vi "STA - Wave V5 Host_Wait_V4.vi"() -> ()   [LabVIEW 2015]
doc: "The continuous acquisition mode tells the FPGA to acquire points indefinitely until a stop command is issued or until an error is encountered (FIFO overflow, module underflow, and so on). \n\nIn this acquisition mode, explicitly call the appropriate rwfm_ConfigTiming VI and set the host application's data buffer to be many times larger than the read size. The examples use a 10X size by default. If the host application's data buffer fills, then the FPGA experiences a FIFO overflow causing the acquisition to stop."
uses:
  <vilib>/LabVIEW Targets/FPGA/cRIO/shared/nicrio_ModuleControls/nicrio_cRIO-9234_ConfigModeRing.ctl
  <vilib>/Platform/TimedLoop/XDataNode/timing_clust.ctl
  <vilib>/Platform/TimedLoop/XDataNode/nitl_modes.ctl
  <vilib>/Platform/TimedLoop/XDataNode/wakeup.ctl
  <vilib>/FPGAPlugInAG/cRIO-9112/niLvFpga_Open_cRIO-9112.vi
  <vilib>/rvi/interface/common/dynamic/niFpgaDynamicAddResources.vi
  <vilib>/Utility/error.llb/Error Cluster From Error Code.vi
  <vilib>/RVI Host/nirviSupport.llb/nirviErrorClusterFromErrorCode.vi
  <vilib>/rvi/errors/niLvFpgaAdjustHostInterfaceError.vi
  <vilib>/FPGAPlugInAG/Dynamic/niLvFpga_Close_Dynamic.vi
  <vilib>/NI/cRIO Wfm/AcqRead(InterleavedSGLs).vi
  <vilib>/rvi/interface/nirviOpenFPGA/nirviOpenFPGA.xnode
  FPGA Bitfiles/STA-WaveformV5_FPGATarget2_[FPGA]DeltaSigMa_sLRIAVfzKK0.lvbitx
  FPGA/[FPGA] DeltaSig Main V5.vi
  <vilib>/rvi/interface/nirviMethod/nirviMethod.xnode
  <vilib>/rvi/interface/nirviCloseFPGA/nirviCloseFPGA.xnode
  <vilib>/Platform/TimedLoop/XDataNode/XDataNode.xnode
  <vilib>/NI/cRIO Wfm/cRIO Wfm.lvlib
  <vilib>/rvi/interface/nirviMethod/StockFPGA_InlinedMethodWaitForSingleIRQ.vi
  <vilib>/FPGAPlugInAG/Dynamic/niLvFpga_WaitOnIrq_Dynamic.vi
  C:/Program Files (x86)/National Instruments/LabVIEW 2015/ProjectTemplates/Source/cRIOWfm/FPGA/[FPGA] SAR Acq Main.vi
  D/Documents/LabVIEW Data/STA - Waveform V0/FPGA Bitfiles/SARAcqMain_9074.lvbitx
  <vilib>/Platform/TimedLoop/XDataNode/XDNodeRunTimeDep.lvlib
panel:
  out "RT Read Side element":u32
  out "RT Write element":u32
  out "Write Side":sgl[][](array[numeric])
  out "transposed array Read Side":sgl[][](array[numeric])
  out "Loop i Read Side":i32
  in  "stop 2":bool
  out "element out Read Side":sgl[](array[numeric])
  out "Write Side out":sgl[](array[numeric])
  in  "Input RTFIFO Create":sgl[](array[numeric])
  in  "Wfm Data":waveform(sgl)[](array[waveform])
  out "Time Measure":dbl
  out "data rate (S/s)":u32
  out "Channel Config":T2(array[cluster]) {"Input Configuration" items=["AC Coupled", "DC Coupled", "IEPE AC Coupled"]}
  in  "Samples per Read":i32=10000
  in  "stop":bool
  out "Waveform Graph Read Side":sgl[](graph)
  out "Buffer Backlog":dbl caption="RT Buffer Backlog [%]" format="%#.2g"
  # "Sampling Info"
  # "Channel Info"
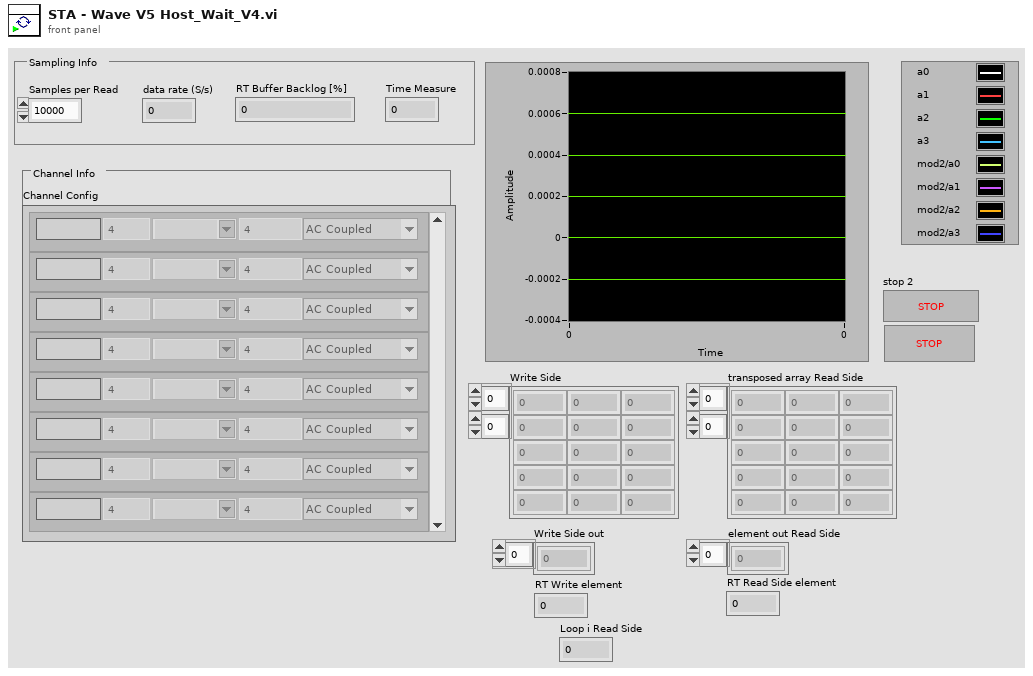
[diagram p1: front panel]
types:
  T1 = typedef "nicrio_cRIO-9234_ConfigModeRing.ctl" = u8
  T2 = cluster{"Channel Name":string, "Sensitivity mV_EU":dbl, "EU":string, "Input Configuration":T1, "dB Ref EU":dbl}[]
  T3 = typedef "XDNodeRunTimeDep.lvlib/timing_clust.ctl" = cluster{"Expected End [f-1]":u64, "Actual End [f-1]":u64, "Finished Late? [f-1]":bool, "Expected End [i-1]":u64, "Actual End [i-1]":u64, "Finished Late? [i-1]":bool, "Expected Start [i]":u64, "Actual Start [i]":u64, "Expected Start [f]":u64, "Actual Start [f]":u64, "Source Name":string, "Structure Name":string, "Period":i64, "Deadline":i64, "Offset":i64, "Start":i64, "Priority":i32, "Timeout":i32, "Mode":T4, "Wakeup Reason":T5, "Error":errorcluster, "Source Type":string, "Secondary Source Type":string, "Global End Time":u64, "Global Start Time":u64, "Frame Duration":u64, "Iteration Duration":u64, "Assigned CPU":i32, "I/O Scan Engine Mode":u32}
  T4 = typedef "XDNodeRunTimeDep.lvlib/nitl_modes.ctl" = enum32{"No Change", "Process missed periods, maintain original phase", "Discard missed periods, maintain original phase", "Process missed periods, ignore original phase", "Discard missed periods, ignore original phase"}
  T5 = typedef "XDNodeRunTimeDep.lvlib/wakeup.ctl" = enum32{"Normal", "Aborted", "Asynchronous wakeup", "Timing source error", "Timed loop error", "Timeout"}
  T6 = typedef "Acquisition and Logging Configuration_Waveform.ctl" = cluster{"Samples per Read":i32, "Number of Reads to Save":i32, "Data File Name":string, "TDMS Properties":T7[], "Number of Channels":i32, "Trigger - RMS Value":dbl, "Trigger - Channel":i32, "Trigger - Time (Minute)":i32, "Channel Config":cluster{"Channel Name":string, "Sensitivity mV_EU":dbl, "EU":string, "Input Configuration":T1, "dB Ref EU":dbl}[], "data rate (S/s)":u32, "Time Measure":dbl}
  T7 = typedef "TDMS Properties.ctl" = cluster{"Name":string, "Value":string}
  T8 = typedef "cRIO Wfm.lvlib/SamplingInfo.ctl" = cluster{"Number of Channels":i32, "Actual Samp Rate":dbl, "Chan Name Array":string[], "EU Chan Array":string[], "dB Ref Chan Array":dbl[]}
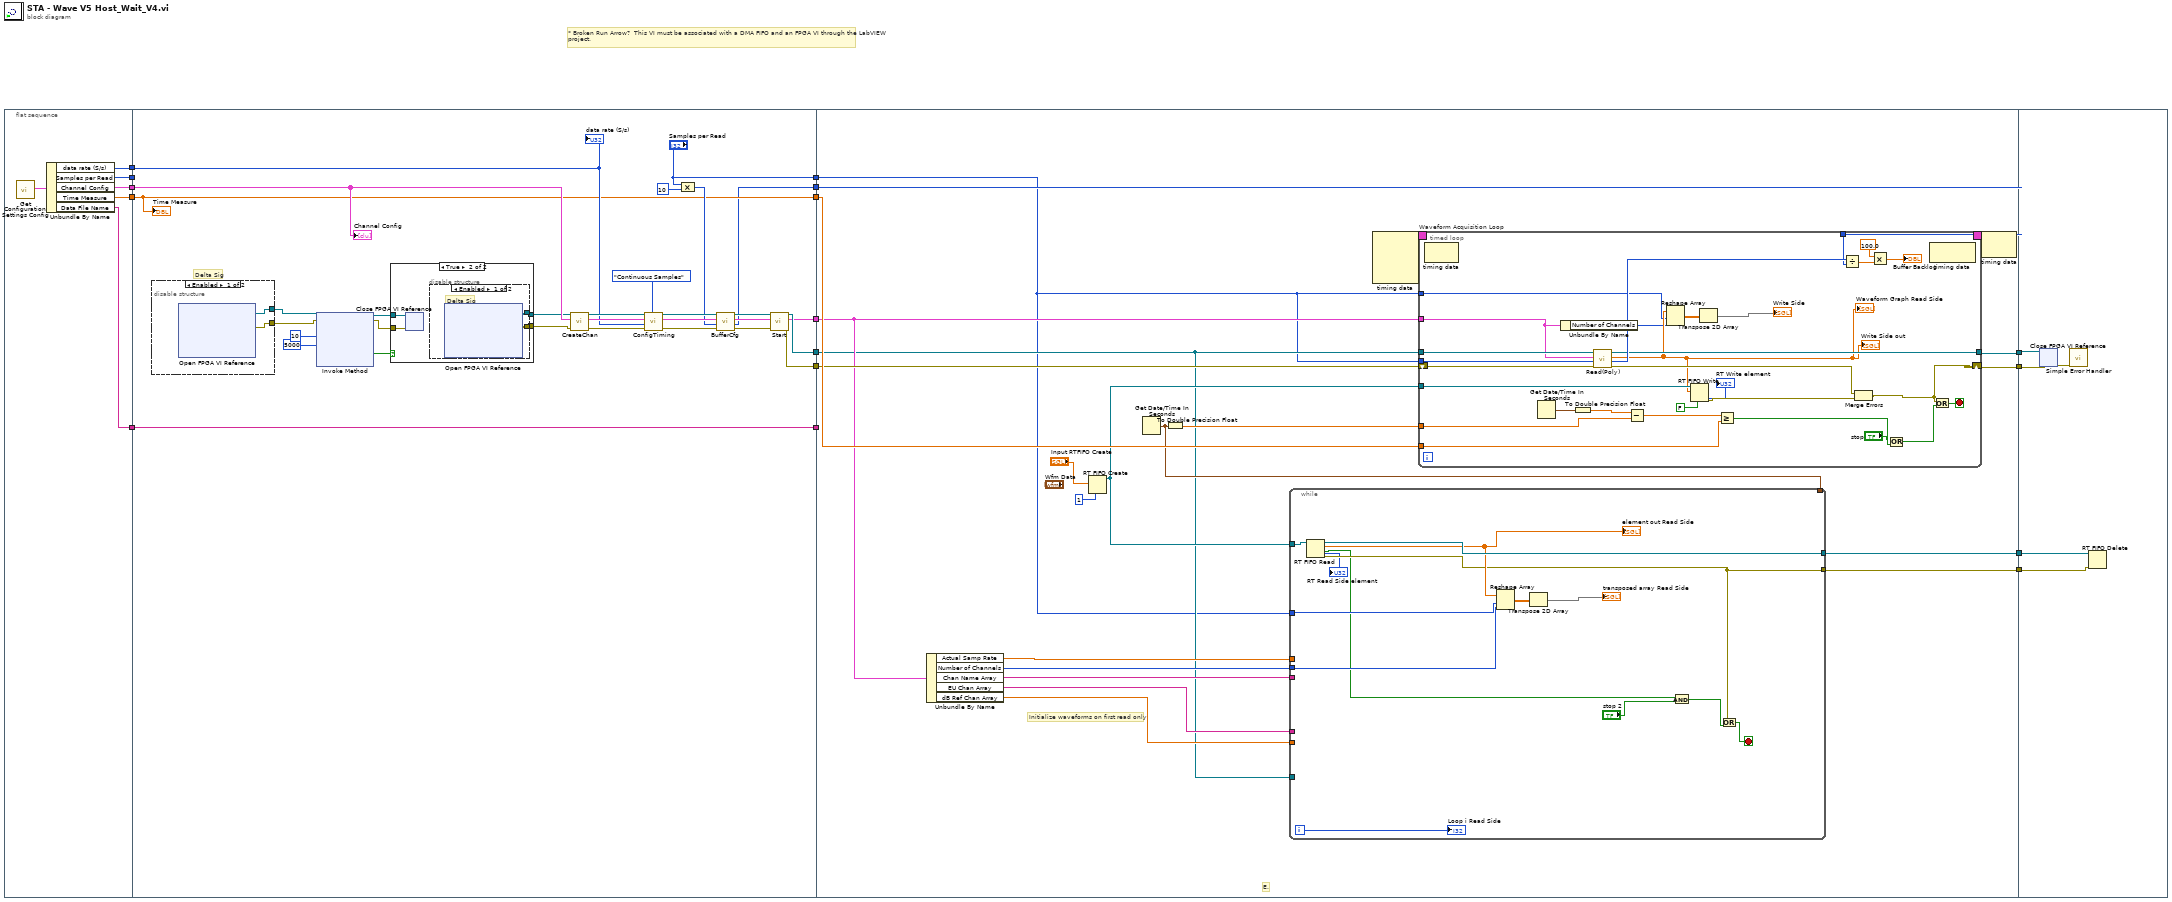
[diagram p0: block diagram]
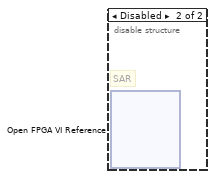
[diagram p2: hidden frame]
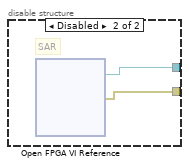
[diagram p4: hidden frame]
diagram:
  # "* Broken Run Arrow?  This VI must be associated with a DMA FIFO and an FPGA VI through the LabVIEW project."
  n1 = flat-sequence {
    tunnel: [w21] -> w16
    tunnel: [w20] -> w15
    tunnel: [w19] -> w14
    tunnel: [w18] -> w13
    tunnel: [w17] -> w4
    tunnel: w16 -> [w34]
    tunnel: w15 -> [_]
    tunnel: w14 -> [w33]
    tunnel: w13 -> [w26]
    tunnel: ["Samples per Read"] -> w12
    tunnel: [w26] -> w11
    tunnel: [w30] -> w10
    tunnel: [w29] -> w9
    tunnel: [w28] -> w8
    tunnel: [w25] -> w7
    tunnel: w4 -> [w24]
    tunnel: [w24] -> w3
    tunnel: w12 -> [w67]
    tunnel: w11 -> [w85]
    tunnel: w10 -> [w68]
    tunnel: w9 -> [w70]
    tunnel: w8 -> [w83]
    tunnel: w7 -> [w84]
    tunnel: [w87] -> w6
    tunnel: [w86] -> w5
    tunnel: w3 -> [_]
    tunnel: [w78] -> w2
    tunnel: [w77] -> w1
    tunnel: w6 -> [w140]
    tunnel: w5 -> [w139]
    tunnel: w2 -> [w138]
    tunnel: w1 -> [w137]
    frame #0 {
      n2 = call "Get Configuration Settings Config.vi"() -> ("Configuration"=w22:T6)  [unwired: 10 in, 1 out]
      n3 = Unbundle By Name(w22) -> ("data rate (S/s)"=w21:u32, "Samples per Read"=w20:i32, "Channel Config"=w19:T2, "Time Measure"=w18:dbl, "Data File Name"=w17:string)
    }
    frame #1 {
      # "Delta Sig"
      n4 = disable-structure shown="Enabled" {
        disable-tunnel: [w54 _] -> w32
        disable-tunnel: [w53 _] -> w31
        frame Enabled {
          n5 = xnode "Open FPGA VI Reference"() -> ("FPGA VI Reference Out"=w54:refnum<k20>, "error out"=w53:errorcluster)  [unwired: 2 in]
        }
        frame Disabled {
          # "SAR"
          n6 = xnode "Open FPGA VI Reference"() -> ("FPGA VI Reference Out"=w56:refnum<k20>, "error out"=w55:errorcluster)  [unwired: 2 in]
        }
      }
      n7 = xnode "Invoke Method"("FPGA VI Reference In"=w32, "error in"=w31, "IRQ Number(s)"=10, "Timeout (ms)"=5000) -> ("FPGA VI Reference Out"=w50:refnum<k20>, "error out"=w51:errorcluster, "Timed Out"=w49:bool)  [unwired: 1 out]
      n8 = case shown="True" w49 {
        tunnel: w50 -> [w58 w62]
        tunnel: w51 -> [w57 w61]
        tunnel: [w58 w60] -> w23
        tunnel: [w57 w59] -> w52
        frame False {
        }
        frame True {
          n9 = xnode "Close FPGA VI Reference"("FPGA VI Reference In"=w62, "error in"=w61) -> ()  [unwired: 1 out]
          n10 = disable-structure shown="Enabled" {
            disable-tunnel: [w64 w66] -> w60
            disable-tunnel: [w63 w65] -> w59
            frame Enabled {
              # "Delta Sig"
              n11 = xnode "Open FPGA VI Reference"() -> ("FPGA VI Reference Out"=w64:refnum<k20>, "error out"=w63:errorcluster)  [unwired: 2 in]
            }
            frame Disabled {
              # "SAR"
              n12 = xnode "Open FPGA VI Reference"() -> ("FPGA VI Reference Out"=w66:refnum<k20>, "error out"=w65:errorcluster)  [unwired: 2 in]
            }
          }
        }
      }
      n13 = call <vilib>:"CreateChan.vi"("Dynamic FPGA Ref"=w23, "Channel Config"=w33, "error in"=w52) -> ("Dynamic FPGA Ref Out"=w40:refnum<k20>, "Sampling Info"=w41:T8, "error out"=w45:errorcluster)  [unwired: 5 in]
      n14 = call <vilib>:"ConfigTiming.vi"("Sample Mode"=enum16{"Finite Samples", "Continuous Samples"}."Continuous Samples", "error in"=w45, "Sample Rate"=w34, "Sampling Info In"=w41, "Dynamic FPGA Ref"=w40) -> ("error out"=w44:errorcluster, "Sampling Info Out"=w43:T8, "Dynamic FPGA Ref Out"=w42:refnum<k20>)  [unwired: 3 in, 1 out]
      n15 = Compound Arithmetic op=MULTIPLY("Samples per Read", 10 ("value")) -> (w38:i32)
      n16 = call <vilib>:"BufferCfg.vi"("error in"=w44, "Buffer Size [Samps per Chan]"=w38, "Sampling Info In"=w43, "Dynamic FPGA Ref"=w42) -> ("error out"=w37:errorcluster, "Buffer Size [Total Samples]"=w25:u32, "Sampling Info Out"=w39:T8, "Dynamic FPGA Ref Out"=w36:refnum<k20>)  [unwired: 4 out]
      n17 = call <vilib>:"Start.vi"("error in"=w37, "Sampling Info In"=w39, "Dynamic FPGA Ref"=w36) -> ("error out"=w28:errorcluster, "Sampling Info Out"=w29:T8, "Dynamic FPGA Ref Out"=w30:refnum<k20>)  [unwired: 6 out]
      "Channel Config" <- w33
      "data rate (S/s)" <- w34
      "Time Measure" <- w26
    }
    frame #2 {
      # "Initialize waveforms on first read only"
      # "E."
      n18 = Unbundle By Name(w70) -> ("Actual Samp Rate"=w73:dbl, "Number of Channels"=w71:i32, "Chan Name Array"=w72:string[], "EU Chan Array"=w74:string[], "dB Ref Chan Array"=w75:dbl[])
      n19 = RT FIFO Create(1:"Input RTFIFO Create", 5:u32 1 ("datapoints in waveform (1)")) -> (8:w79:refnum<k33>)  [unwired: 6 in, 2 out]
      n20 = Get Date/Time In Seconds() -> (seconds since 1Jan1904=w69:timestamp)
      n21 = To Double Precision Float(number=w69) -> (double precision float=w88:dbl)
      n22 = while {
        tunnel: w79 -> [w102]
        tunnel: [w101] -> w78
        tunnel: [w94] -> w77
        tunnel: w75 -> [_]
        tunnel: w74 -> [_]
        tunnel: w73 -> [_]
        tunnel: w72 -> [_]
        tunnel: w71 -> [w96]
        tunnel: w67 -> [w95]
        tunnel: w69 -> [_]
        tunnel: w68 -> [_]
        i -> [w99]
        stop <- w100 stop-if-true
        n23 = RT FIFO Read(0:w102) -> (7:→"RT Read Side element":u32, 8:w101:refnum<k33>, 9:w97:sgl[], 10:w90:bool, 11:w94:errorcluster)  [unwired: 3 in]
        "element out Read Side" <- w97
        n24 = Reshape Array(w97, w95, w96) -> (w98:sgl[][])
        n25 = Transpose 2D Array(2D array=w98) -> (transposed array=→"transposed array Read Side":sgl[][])
        n26 = And(x=w90, y="stop 2") -> (x .and. y?=w89:bool)
        n27 = Or(x=w94, y=w89) -> (x .or. y?=w100:bool)
        "Loop i Read Side" <- w99
      }
      n28 = node-c288() -> (w81:T3)  [unwired: 4 in]
      n29 = timed-loop "Waveform Acquisition Loop" {
        tunnel: [w126] -> w87
        shift-right: [w124] -> w86
        shift-left: w83 -> [w132]
        tunnel: w88 -> [w117]
        tunnel: w85 -> [w116]
        tunnel: w68 -> [w115]
        tunnel: w70 -> [w106]
        tunnel: w67 -> [w114]
        tunnel: w84 -> [w113]
        tunnel: w79 -> [w112]
        timing: w81 -> [_]
        timing-out: [_] -> w80
        tunnel: w67 -> [w107]
        stop <- w127 stop-if-true
        n30 = node-c288() -> ()  [unwired: 1 in, 1 out]
        n31 = Get Date/Time In Seconds() -> (seconds since 1Jan1904=w119:timestamp)
        n32 = Unbundle By Name(w106) -> ("Number of Channels"=w105:i32)
        n33 = To Double Precision Float(number=w119) -> (double precision float=w118:dbl)
        n34 = call-poly <vilib>:"Read(Poly).vi"("error in"=w132, "Samps Read per Chan"=w114, "Sampling Info"=w106, "Dynamic FPGA Ref"=w115) -> ("error out"=w125:errorcluster, "Samples Remaining"=w131:u32, "Data"=w108:sgl[], "Dynamic FPGA Ref Out"=w126:refnum<k20>)  [unwired: 4 in]
        "Waveform Graph Read Side" <- w108
        "Write Side out" <- w108
        n35 = Subtract(x=w118, y=w117) -> (x-y=w120:dbl)
        n36 = Reshape Array(w108, w107, w105) -> (w110:sgl[][])
        n37 = RT FIFO Write(0:w112, 1:w108, 5:FALSE ("overwrite on timeout (T)")) -> (7:→"RT Write element":u32, 11:w111:errorcluster)  [unwired: 2 in, 2 out]
        n38 = Transpose 2D Array(2D array=w110) -> (transposed array=→"Write Side":sgl[][])
        n39 = Greater Or Equal?(x=w120, y=w116) -> (x >= y?=w123:bool)
        n40 = Divide(x=w131, y=w113) -> (x/y=w130:dbl)
        n41 = Merge Errors(w125, w111) -> (w124:errorcluster)
        n42 = Multiply(x=100.0, y=w130) -> (x*y=→"Buffer Backlog":dbl)
        n43 = Or(x="stop", y=w123) -> (x .or. y?=w121:bool)
        n44 = node-c288() -> ()  [unwired: 1 in, 1 out]
        n45 = Or(x=w124, y=w121) -> (x .or. y?=w127:bool)
      }
      n46 = node-c288(w80) -> ()  [unwired: 1 out]
    }
    frame #3 {
      n47 = xnode "Close FPGA VI Reference"("FPGA VI Reference In"=w140, "error in"=w139) -> ("error out"=w141:errorcluster)
      n48 = call <vilib>:"Simple Error Handler.vi"("error in (no error)"=w141) -> ()  [unwired: 1 in, 8 out]
      n49 = RT FIFO Delete(0:w138, 3:w137) -> ()  [unwired: 1 in, 1 out]
    }
  }
